vi "wait4noti.vi"(8 "error in (no error)":errorcluster, 10 "N":i32=1, 11 "notifier":refnum<notifier>) -> (0 "error out":errorcluster, 3 "notifier out":refnum<notifier>)   [LabVIEW 2020]
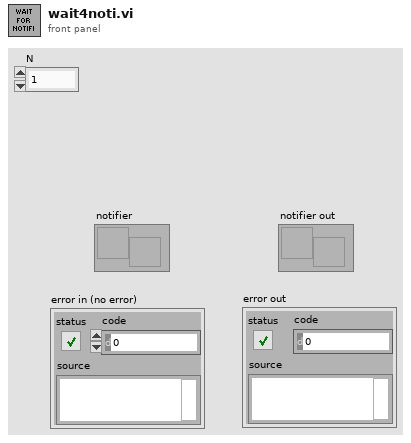
[diagram p1: front panel]
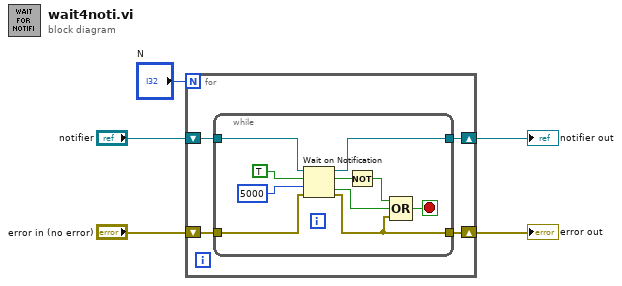
[diagram p0: block diagram]
diagram:
  n1 = for {
    N: "N" -> [_]
    shift-right: [w7] -> w3
    shift-left: "notifier" -> [w9]
    shift-right: [w8] -> w4
    shift-left: "error in (no error)" -> [w6]
    n2 = while {
      tunnel: [w19] -> w7
      tunnel: w9 -> [w16]
      tunnel: [w11] -> w8
      tunnel: w6 -> [w15]
      stop <- w10 stop-if-true
      n3 = Wait on Notification(notifier=w16, ignore previous (F)=TRUE, timeout in ms (-1)=5000, error in (no error)=w15) -> (notifier out=w19:refnum<notifier>, notification=w14:bool, timed out?=w12:bool, error out=w11:errorcluster)
      n4 = Not(x=w14) -> (.not. x?=w13:bool)
      n5 = Compound Arithmetic op=OR(w13, w12, w11) -> (w10:bool)
    }
  }
  "error out" <- w4
  "notifier out" <- w3
